vi "Interface Write.vi"(8 "error in":errorcluster, 9 "timeout":i32=10000, 10 "data":u8[](array[numeric]), 11 "interface in":refnum<class "Network Interface.lvclass">) -> (0 "error out":errorcluster, 1 "timed out?":bool, 3 "interface out":refnum<class "Network Interface.lvclass">)   [LabVIEW 2021, in "Network Interface.lvclass"]
doc: "This provides an interface for writing to a network bus."
uses:
  Network Interface.lvclass
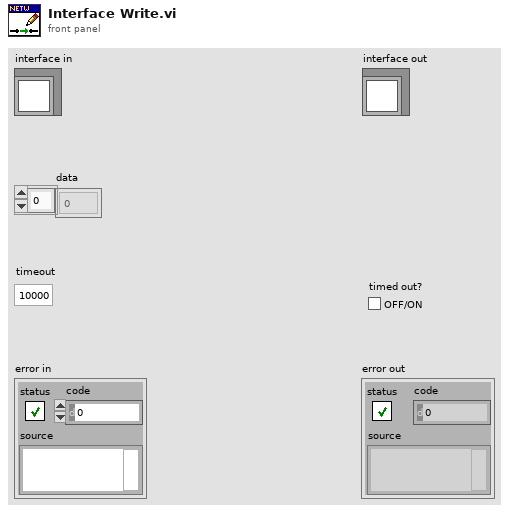
[diagram p1: front panel]
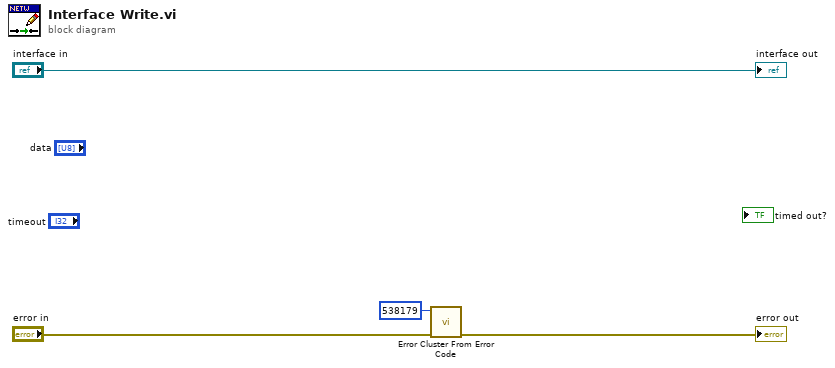
[diagram p0: block diagram]
diagram:
  n1 = call <vilib>:"Error Cluster From Error Code.vi"("error in (no error)"="error in", "error code (0)"=538179) -> ("error out"=→"error out":errorcluster)  [unwired: 7 in]
  "interface out" <- "interface in"
